vi "error_collect.vi"(10 "error in (no error)":errorcluster caption="错误输入（无错误）") -> (2 "error IO":errorcluster)   [LabVIEW 2014]
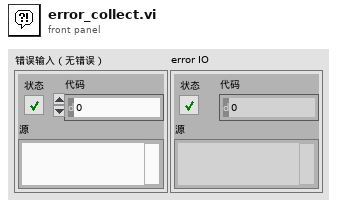
[diagram p1: front panel]
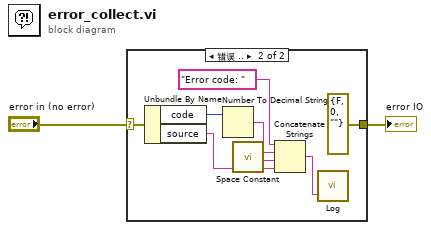
[diagram p0: block diagram]
diagram:
  n1 = case shown="错误 .." "error in (no error)" {
    selector: "error in (no error)" -> [w3 w11]
    tunnel: [w3 errorcluster {"status"=FALSE, "code"=0, "source"=""}] -> w1
    frame No Error {
    }
    frame Error {
      n2 = Unbundle By Name(w11) -> ("code"=w5:i32, "source"=w10:string)
      n3 = Number To Decimal String(number=w5) -> (decimal integer string=w4:string)  [unwired: 1 in]
      n4 = call <vilib>:"Space Constant.vi"() -> ("String"=w6:string)
      n5 = Concatenate Strings("Error code: " ("字符串"), w4, w6, w10) -> (w8:string)
      n6 = call "Log.vi"("Data"=w8) -> ()  [unwired: 3 in]
    }
  }
  "error IO" <- w1
